vi "FetchServoResults.vi"(8 "error in":errorcluster, 10 "rfsgSession":refnum<k15>, 11 "ServoSessionIn":u32) -> (0 "error out":errorcluster, 2 "Servo Results":T1={"Final Input Power (dBm)"=0.05, "Final Output Power (dBm)"=0.05, "Calculated Dut Gain (dB)"=0.05, "Servo Trace"=[]}, 3 "ServoSessionOut":u32)   [LabVIEW 2016, in "Power Servo.lvlib"]
uses:
  Power Servo.lvlib
  Type Definitions/ServoResult.ctl
  <userlib>/_NI Power Servoing IP/HostRdl/NI Power Servoing IP New (Host).lvlib
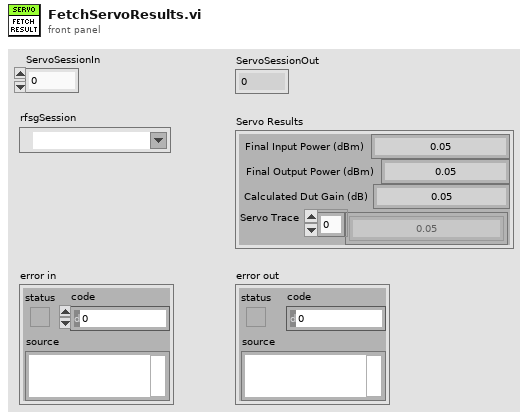
[diagram p1: front panel]
types:
  T1 = typedef "Power Servo.lvlib/ServoResult.ctl" = cluster{"Final Input Power (dBm)":dbl, "Final Output Power (dBm)":dbl, "Calculated Dut Gain (dB)":dbl, "Servo Trace":dbl[]}
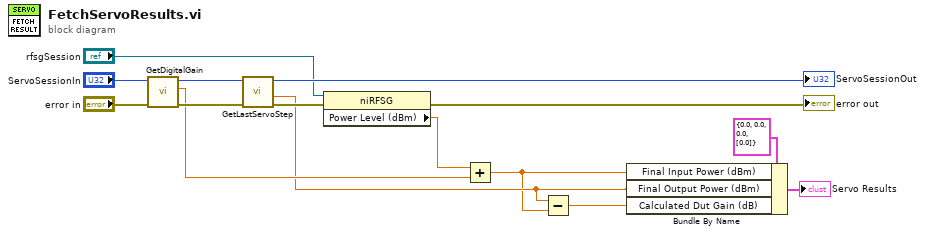
[diagram p0: block diagram]
diagram:
  n1 = call <userlib>:"GetDigitalGain.vi"("error in"="error in", "SessionHandleIn"="ServoSessionIn") -> ("error out"=w12:errorcluster, "DigitalGainDB"=w6:dbl, "SessionHandleOut"=w13:u32)  [unwired: 6 in, 1 out]
  n2 = call <userlib>:"GetLastServoStep.vi"("error in"=w12, "SessionHandleIn"=w13) -> ("error out"=w9:errorcluster, "measurement_level_dBm"=w4:dbl, "SessionHandleOut"=→"ServoSessionOut":u32)  [unwired: 6 in, 1 out]
  n3 = property class="niRFSG"(reference="rfsgSession", error in=w9) -> (error out=→"error out":errorcluster, "Power Level (dBm)"=w7:dbl)  [unwired: 1 out]
  n4 = Add(x=w7, y=w6) -> (x+y=w3:dbl)
  n5 = Subtract(x=w4, y=w3) -> (x-y=w2:dbl)
  n6 = Bundle By Name(cluster=T1 {"Final Input Power (dBm)"=0.0, "Final Output Power (dBm)"=0.0, "Calculated Dut Gain (dB)"=0.0, "Servo Trace"=[0.0]} ("Servo Result"), "Final Input Power (dBm)"=w3, "Final Output Power (dBm)"=w4, "Calculated Dut Gain (dB)"=w2) -> (→"Servo Results":T1)
